vi "Calculate Distribution Sizes.vi"(7 "size":i16=500, 8 "error in (no error)":errorcluster, 10 "Visible":bool[](array[boolean]), 11 "Container in":refnum<class "Divider.lvclass">) -> (0 "error out":errorcluster, 2 "Start":i16[](array[numeric]), 3 "Container out":refnum<class "Divider.lvclass">)   [LabVIEW 2021, in "Divider.lvclass"]
doc: "Copyright 2018, Wiebe Walstra, wiebe@carya.nl."
uses:
  Divider.lvclass
  Divider.lvclass/Divider.ctl
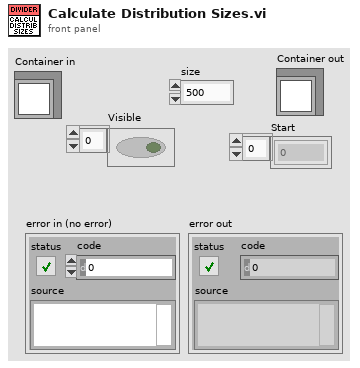
[diagram p1: front panel]
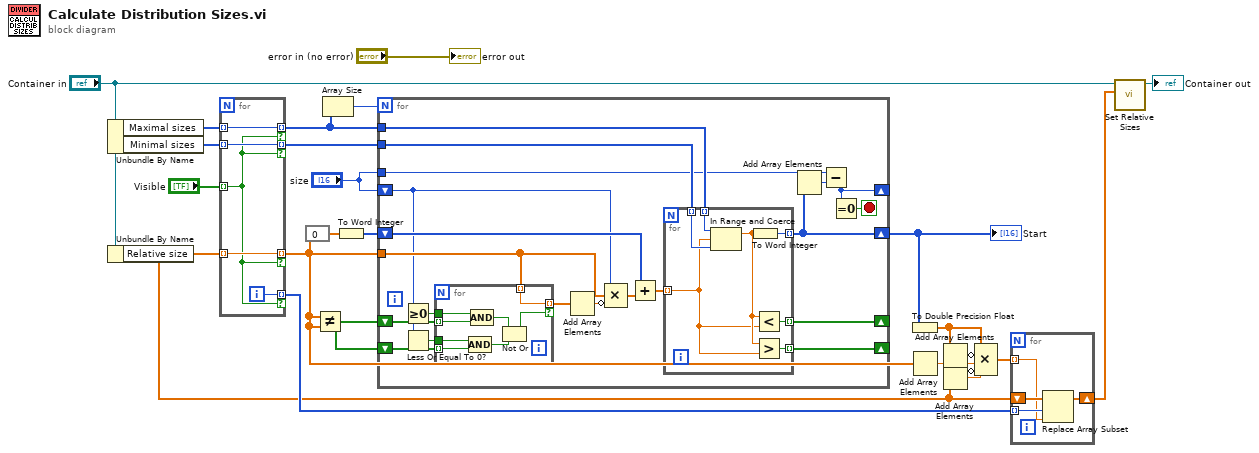
[diagram p0: block diagram]
diagram:
  n1 = Unbundle By Name("Container in") -> ("Maximal sizes"=w18:i16[], "Minimal sizes"=w16:i16[])
  n2 = Unbundle By Name("Container in") -> ("Relative size"=w7:dbl[])
  n3 = for {
    tunnel: [w28] -> w19 mode=indexing if=w24
    tunnel: w18 -> [w28] mode=indexing
    tunnel: [w27] -> w17 mode=indexing if=w24
    tunnel: w16 -> [w27] mode=indexing
    tunnel: [w26] -> w8 mode=indexing if=w24
    tunnel: w7 -> [w26] mode=indexing
    tunnel: "Visible" -> [w24] mode=indexing
    tunnel: [w25] -> w13 mode=indexing if=w24
    i -> [w25]
  }
  n4 = expression code="0"(w8) -> (w22:dbl[])
  n5 = Not Equal?(x=w8, y=w8) -> (x != y?=w21:bool[])
  n6 = Array Size(array=w19) -> (size(s)=w23:i32)
  n7 = To Word Integer(number=w22) -> (16bit integer=w14:i16[])
  n8 = for {
    N: w23 -> [_]
    tunnel: w19 -> [w45]
    tunnel: w17 -> [w44]
    shift-right: [w36] -> w2
    shift-left: w14 -> [w40]
    shift-right: [w43] -> _
    shift-left: w21 -> [w48]
    shift-right: [w42] -> _
    shift-left: w21 -> [w47]
    tunnel: w8 -> [w39]
    tunnel: "size" -> [w34]
    shift-right: [w29] -> _
    shift-left: "size" -> [w31]
    stop <- w33 stop-if-true
    n9 = Greater Or Equal To 0?(x=w31) -> (x >= 0?=w32:bool)
    n10 = Less Or Equal To 0?(x=w31) -> (x <= 0?=w30:bool)
    n11 = for {
      tunnel: w48 -> [w56] mode=indexing
      tunnel: w47 -> [w55] mode=indexing
      tunnel: w39 -> [w54] mode=indexing
      tunnel: [w54] -> w46 mode=indexing if=w53
      tunnel: w32 -> [w51]
      tunnel: w30 -> [w49]
      n12 = Compound Arithmetic op=AND(w49, w55) -> (w50:bool)
      n13 = Compound Arithmetic op=AND(w51, w56) -> (w52:bool)
      n14 = Not Or(1:w50, 2:w52) -> (0:w53:bool)
    }
    n15 = Add Array Elements(numeric array=w46) -> (sum=w37:dbl)
    n16 = Compound Arithmetic op=MULTIPLY(w31, w39, invert w37) -> (w38:dbl[])
    n17 = Add(x=w40, y=w38) -> (x+y=w41:dbl[])
    n18 = for {
      tunnel: w41 -> [w59] mode=indexing
      tunnel: w45 -> [w63] mode=indexing
      tunnel: w44 -> [w62] mode=indexing
      tunnel: [w57] -> w36 mode=indexing
      tunnel: [w61] -> w43 mode=indexing
      tunnel: [w58] -> w42 mode=indexing
      n19 = In Range and Coerce(upper limit=w63, x=w59, lower limit=w62) -> (coerced(x)=w60:dbl)  [unwired: 1 out]
      n20 = To Word Integer(number=w60) -> (16bit integer=w57:i16)
      n21 = Less?(x=w60, y=w59) -> (x < y?=w61:bool)
      n22 = Greater?(x=w60, y=w59) -> (0:w58:bool)
    }
    n23 = Add Array Elements(numeric array=w36) -> (sum=w35:i16)
    n24 = Subtract(x=w34, y=w35) -> (x-y=w29:i16)
    n25 = Equal To 0?(x=w29) -> (x = 0?=w33:bool)
  }
  "Start" <- w2
  n26 = To Double Precision Float(number=w2) -> (double precision float=w1:dbl[])
  n27 = Add Array Elements(numeric array=w8) -> (sum=w5:dbl)
  n28 = Add Array Elements(numeric array=w1) -> (sum=w3:dbl)
  n29 = Add Array Elements(numeric array=w7) -> (sum=w6:dbl)
  n30 = Compound Arithmetic op=MULTIPLY(w1, invert w3, w5, invert w6) -> (w4:dbl[])
  n31 = for {
    tunnel: w13 -> [w65] mode=indexing
    shift-right: [w66] -> w11
    shift-left: w7 -> [w67]
    tunnel: w4 -> [w64] mode=indexing
    n32 = Replace Array Subset(array=w67, new element=w64, index=w65) -> (w66:dbl[])
  }
  n33 = call "Set Relative Sizes.vi"("Relative sizes"=w11, "Divider in"="Container in") -> ("Divider out"=→"Container out":refnum<class "Divider.lvclass">)  [unwired: 8 in, 1 out]
  "error out" <- "error in (no error)"
